vi "数组行列读取.vi"(8 "错误输入（无错误）":errorcluster, 11 "引用":refnum<vi>) -> (0 "错误输出":errorcluster, 2 "行列":T1, 3 "引用输出":refnum<vi>)   [LabVIEW 2014, in "表格.lvlib"]
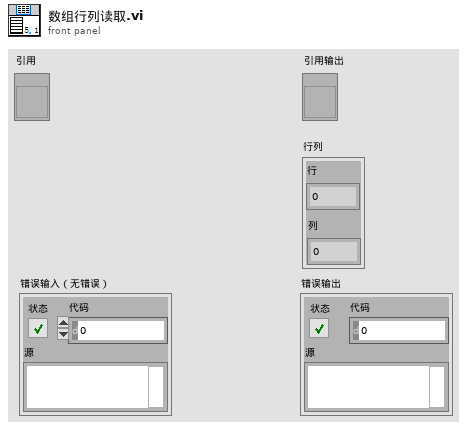
[diagram p1: front panel]
types:
  T1 = typedef "行列.ctl" = cluster{"行":i32, "列":i32}
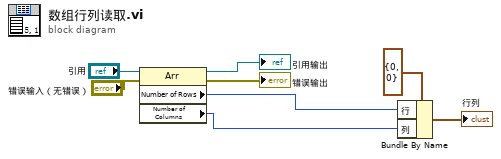
[diagram p0: block diagram]
diagram:
  n1 = property class="Arr"(reference="引用", error in="错误输入（无错误）") -> (reference out=→"引用输出":refnum<vi>, error out=→"错误输出":errorcluster, "Number of Rows"=w3:u32, "Number of Columns"=w2:u32)
  n2 = Bundle By Name(cluster=T1 {"行"=0, "列"=0} ("行列"), "行"=w3, "列"=w2) -> (→"行列":T1)
